vi "Read DATA.vi"(11 "OscillationDetector in":refnum<class "OscillationDetector.lvclass">) -> (1 "DATA PERIOD":T1, 2 "DATA N":T1, 4 "UPPER TH":dbl, 6 "LOWER TH":dbl)   [LabVIEW 2019, in "OscillationDetector.lvclass"]
uses:
  OscillationDetector.lvclass
  DATA Oscill.ctl
  OscillationDetector.lvclass/OscillationDetector.ctl
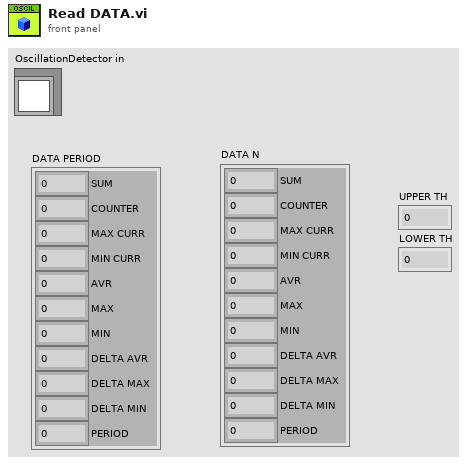
[diagram p1: front panel]
types:
  T1 = typedef "DATA Oscill.ctl" = cluster{"SUM":dbl, "COUNTER":dbl, "MAX CURR":dbl, "MIN CURR":dbl, "AVR":dbl, "MAX":dbl, "MIN":dbl, "DELTA AVR":dbl, "DELTA MAX":dbl, "DELTA MIN":dbl, "PERIOD":dbl}
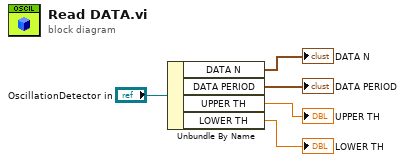
[diagram p0: block diagram]
diagram:
  n1 = Unbundle By Name("OscillationDetector in") -> ("DATA N"=→"DATA N":T1, "DATA PERIOD"=→"DATA PERIOD":T1, "UPPER TH"=→"UPPER TH":dbl, "LOWER TH"=→"LOWER TH":dbl)
